vi "EXCOM-TCP-READ.vi"(6 "Error In":errorcluster, 9 "connection ID":refnum<k5>) -> (0 "Error Out":errorcluster, 1 "Response":string, 3 "CID Out":refnum<k5>)   [LabVIEW 2019]
panel:
  out "Length":i32
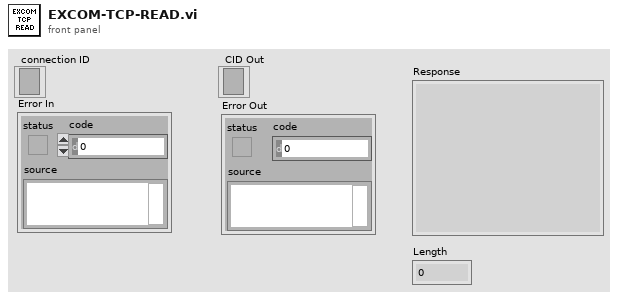
[diagram p1: front panel]
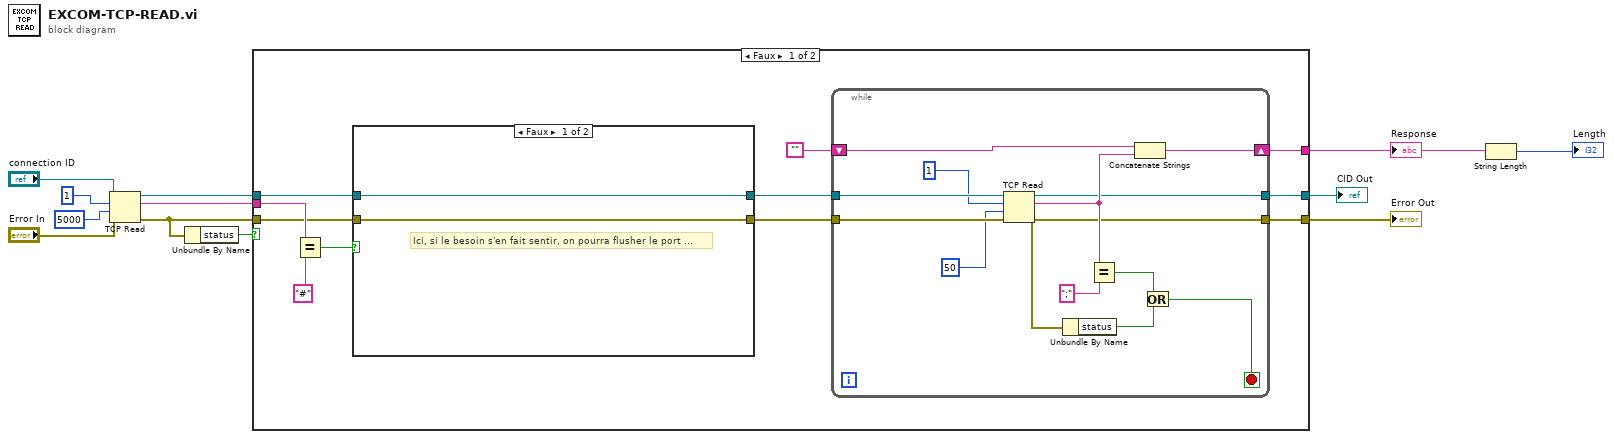
[diagram p0: block diagram]
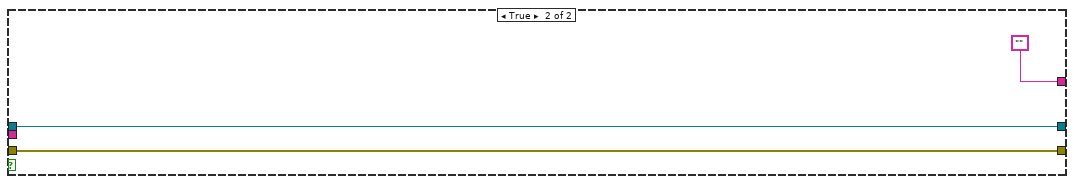
[diagram p3: hidden frame]
diagram:
  n1 = TCP Read(connection ID="connection ID", bytes to read=1, error in (no error)="Error In", 9:5000 ("timeout ms (25000)")) -> (connection ID out=w7:refnum<k5>, data out=w8:string, error out=w6:errorcluster)  [unwired: 1 in]
  n2 = Unbundle By Name(w6) -> ("status"=w9:bool)
  n3 = case shown="Faux" w9 {
    tunnel: w8 -> [w23 _]
    tunnel: w7 -> [w20 w42]
    tunnel: w6 -> [w19 w41]
    tunnel: [w15 ""] -> w3
    tunnel: [w14 w41] -> w5
    tunnel: [w13 w42] -> w4
    frame False {
      n4 = Equal?(x=w23, y="#") -> (x = y?=w21:bool)
      n5 = case shown="Faux" w21 {
        tunnel: w20 -> [w25 w27]
        tunnel: w19 -> [w24 w26]
        tunnel: [w25 w27] -> w18
        tunnel: [w24 w26] -> w17
        frame False {
          # "Ici, si le besoin s'en fait sentir, on pourra flusher le port ..."
        }
        frame True {
        }
      }
      n6 = while {
        tunnel: w18 -> [w40]
        tunnel: w17 -> [w39]
        shift-right: [w32] -> w15
        shift-left: "" -> [w33]
        tunnel: [w28] -> w14
        tunnel: [w31] -> w13
        stop <- w35 stop-if-true
        n7 = TCP Read(connection ID=w40, bytes to read=1, error in (no error)=w39, 9:50 ("timeout ms (25000)")) -> (connection ID out=w31:refnum<k5>, data out=w34:string, error out=w28:errorcluster)  [unwired: 1 in]
        n8 = Unbundle By Name(w28) -> ("status"=w36:bool)
        n9 = Equal?(x=w34, y=";") -> (x = y?=w37:bool)
        n10 = Concatenate Strings(w33, w34) -> (w32:string)
        n11 = Or(x=w37, y=w36) -> (x .or. y?=w35:bool)
      }
    }
    frame True {
    }
  }
  "Response" <- w3
  "Error Out" <- w5
  "CID Out" <- w4
  n12 = String Length(string=w3) -> (length=→"Length":i32)
